vi "0.4_кВ_В2.vi"(9 "Time delay":dbl, 10 "Авария ВВОД 1":bool) -> (1 "АВР\nВВОД 2":bool, 2 "Амперметр 0,4 кВ ВВОД 2":dbl(knob) scale=0.0..630.0, 3 "Вольтметр 0,4 кВ ВВОД 2":i64(knob) scale=340.0..420.0)   [LabVIEW 2016]
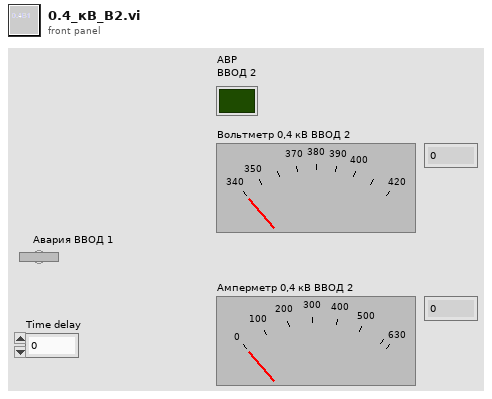
[diagram p1: front panel]
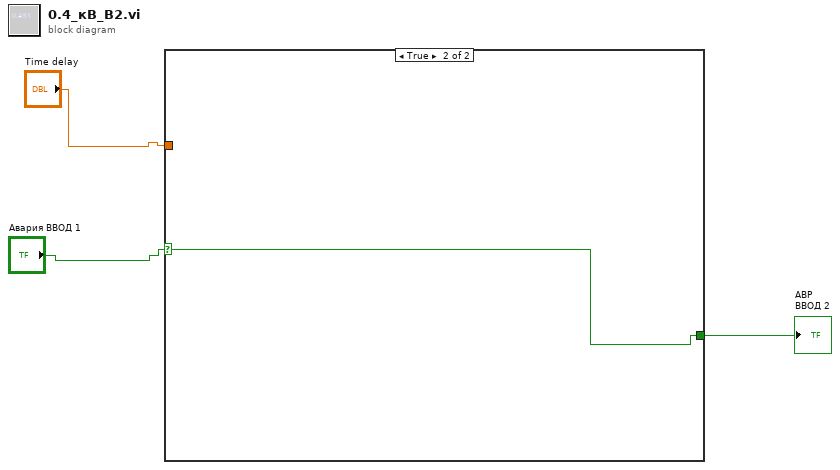
[diagram p0: block diagram]
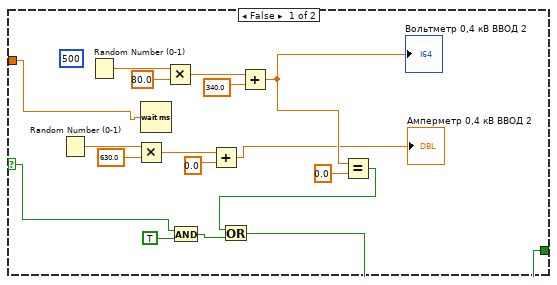
[diagram p2: hidden frame]
diagram:
  n1 = case shown="True" "Авария ВВОД 1" {
    selector: "Авария ВВОД 1" -> [w6 w21]
    tunnel: "Time delay" -> [w5 _]
    tunnel: [w4 w21] -> w1
    frame False {
      (unwired) u32 500 ("milliseconds to wait")
      n2 = Random Number (0-1)() -> (number: 0 to 1=w13:dbl)
      n3 = Random Number (0-1)() -> (number: 0 to 1=w17:dbl)
      n4 = Multiply(x=w13, y=630.0) -> (x*y=w11:dbl)
      n5 = Wait (ms)(milliseconds to wait=w5) -> ()  [unwired: 1 out]
      n6 = Multiply(x=w17, y=80.0) -> (x*y=w15:dbl)
      n7 = And(x=w6, y=TRUE) -> (x .and. y?=w8:bool)
      n8 = Add(x=w11, y=0.0) -> (x+y=→"Амперметр 0,4 кВ ВВОД 2":dbl)
      n9 = Add(x=w15, y=340.0) -> (x+y=w20:dbl)
      "Вольтметр 0,4 кВ ВВОД 2" <- w20
      n10 = Equal?(x=w20, y=0.0) -> (x = y?=w7:bool)
      n11 = Or(x=w7, y=w8) -> (x .or. y?=w4:bool)
    }
    frame True {
    }
  }
  "АВР\nВВОД 2" <- w1
